vi "Set Initialization Data - File mainpulate.vi"(8 "error in":errorcluster, 11 "UI SmarAct in":refnum<class "UI SmarAct.lvclass">) -> (0 "error out":errorcluster, 3 "UI SmarAct out":refnum<class "UI SmarAct.lvclass">)   [LabVIEW 2024, in "UI SmarAct.lvclass"]
doc: "In this VI you can set the initialization data of a statically-linked subWorker."
uses:
  UI SmarAct.lvclass
  File manipulate/Initialization Data.ctl
  File manipulate/Response Cases.ctl
  UI SmarAct.lvclass/UI SmarAct.ctl
  File manipulate/File manipulate.lvclass
  C:/Program Files (x86)/National Instruments/LabVIEW 2024/vi.lib/addons/_Workers/Library/Classes/Worker/Worker.lvclass
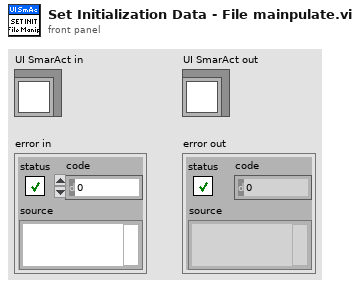
[diagram p1: front panel]
types:
  T1 = typedef "File manipulate.lvclass/Initialization Data.ctl" = cluster{"Response Cases":T2}
  T2 = typedef "File manipulate.lvclass/Response Cases.ctl" = cluster{"Placeholder - Can be deleted":string}
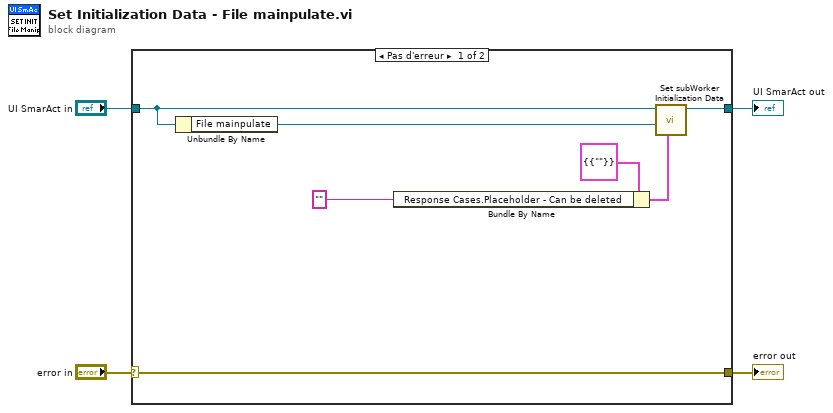
[diagram p0: block diagram]
diagram:
  n1 = case shown="Pas d'erreur" "error in" {
    selector: "error in" -> [w11 w13]
    tunnel: [w11 w13] -> w3
    tunnel: [w9 w12] -> w2
    tunnel: "UI SmarAct in" -> [w8 w12]
    frame No Error {
      n2 = Unbundle By Name(w8) -> ("File mainpulate"=w10:refnum<class "File manipulate.lvclass">)
      n3 = Bundle By Name(cluster=T1 {"Response Cases"={"Placeholder - Can be deleted"=""}} ("Initialization Data"), "Response Cases.Placeholder - Can be deleted"="" ("Placeholder")) -> (w6:T1)
      n4 = call-dynamic "Set subWorker Initialization Data.vi"("Initialization Data"=w6, "subWorker"=w10, "Worker"=w8) -> ("Worker out"=w9:refnum<class "UI SmarAct.lvclass">)  [unwired: 8 in]
    }
    frame Error {
    }
  }
  "error out" <- w3
  "UI SmarAct out" <- w2
